vi "FPGA_main.vi"() -> ()   [LabVIEW 2016]
uses:
  <vilib>/Platform/TimedLoop/XDataNode/timing_clust.ctl
  <vilib>/Platform/TimedLoop/XDataNode/nitl_modes.ctl
  <vilib>/Platform/TimedLoop/XDataNode/wakeup.ctl
  FPGA_states.ctl
  <vilib>/rvi/Emulation/niFpgaSctlEmulationGetInTimedLoop.vi
  <vilib>/rvi/Emulation/niFpgaEmulationReportErrorSimple.vi
  <vilib>/rvi/Emulation/niFpgaGetClockAttributes.vi
  <vilib>/rvi/Emulation/niFpgaCriticalErrorInLSC.vi
  <vilib>/rvi/interface/RandomDataEmulation/niFpgaRandomDataHandleErrors.vi
  <vilib>/Platform/TimedLoop/XDataNode/XDataNode.xnode
  <vilib>/rvi/DataTransferAndStorage/Container/XNode/niFpgaContainer.xnode
  <vilib>/rvi/interface/RandomDataEmulation/nirviRandomDataFpgaReadWriteTemplate.vi
  <vilib>/Platform/TimedLoop/XDataNode/XDNodeRunTimeDep.lvlib
  <instrlib>/_niInstr/Basic Elements/v1/FPGA/niInstr Basic Elements v1 FPGA.lvlib
panel:
  in  "BatchSize":u64
  in  "StartTransfer":bool
  out "Count":u64
  out "Iteration":i32
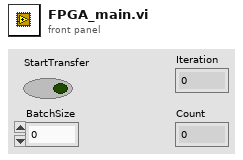
[diagram p1: front panel]
types:
  T1 = typedef "FPGA_states.ctl" = enum16{"Idle", "Flush_FIFO", "CountUp&Transfer"}
  T2 = typedef "XDNodeRunTimeDep.lvlib/timing_clust.ctl" = cluster{"Expected End [f-1]":u64, "Actual End [f-1]":u64, "Finished Late? [f-1]":bool, "Expected End [i-1]":u64, "Actual End [i-1]":u64, "Finished Late? [i-1]":bool, "Expected Start [i]":u64, "Actual Start [i]":u64, "Expected Start [f]":u64, "Actual Start [f]":u64, "Source Name":string, "Structure Name":string, "Period":i64, "Deadline":i64, "Offset":i64, "Start":i64, "Priority":i32, "Timeout":i32, "Mode":T3, "Wakeup Reason":T4, "Error":errorcluster, "Source Type":string, "Secondary Source Type":string, "Global End Time":u64, "Global Start Time":u64, "Frame Duration":u64, "Iteration Duration":u64, "Assigned CPU":i32, "I/O Scan Engine Mode":u32}
  T3 = typedef "XDNodeRunTimeDep.lvlib/nitl_modes.ctl" = enum32{"No Change", "Process missed periods, maintain original phase", "Discard missed periods, maintain original phase", "Process missed periods, ignore original phase", "Discard missed periods, ignore original phase"}
  T4 = typedef "XDNodeRunTimeDep.lvlib/wakeup.ctl" = enum32{"Normal", "Aborted", "Asynchronous wakeup", "Timing source error", "Timed loop error", "Timeout"}
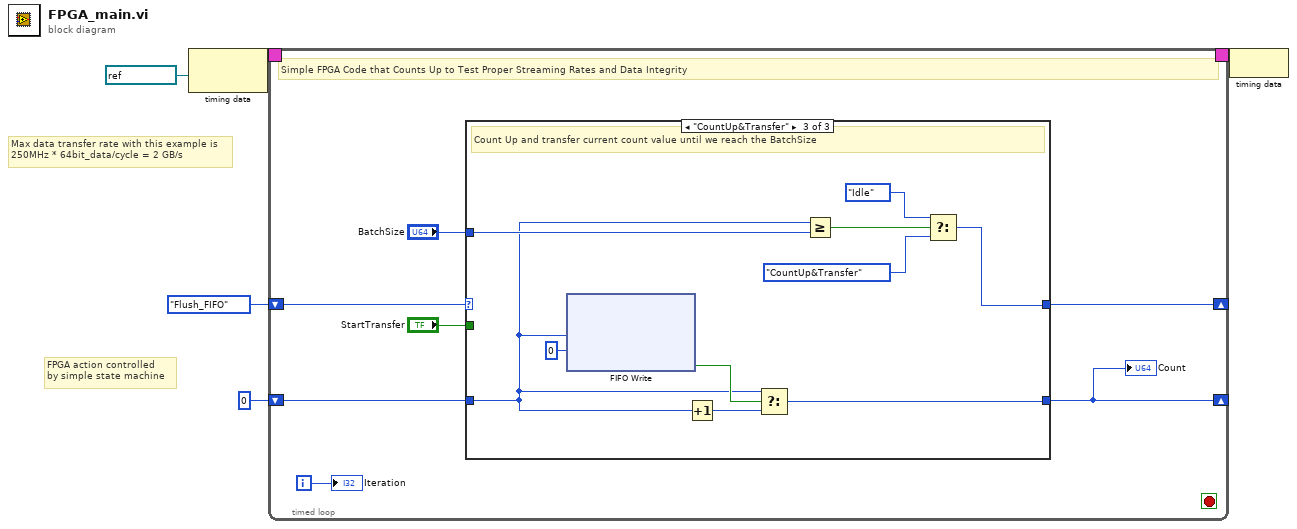
[diagram p0: block diagram]
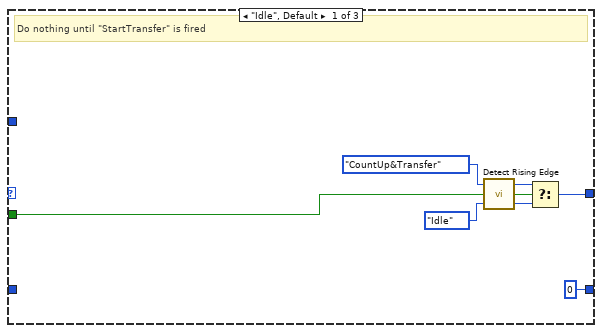
[diagram p2: hidden frame]
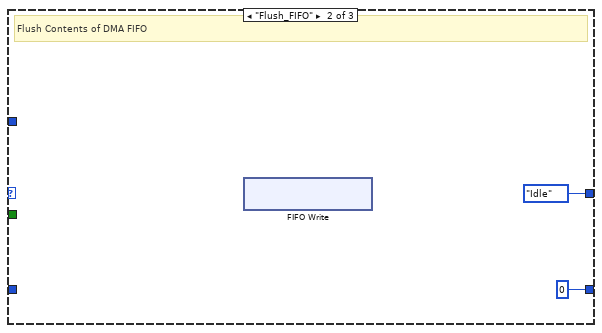
[diagram p3: hidden frame]
diagram:
  # "Max data transfer rate with this example is\n250MHz * 64bit_data/cycle = 2 GB/s"
  # "FPGA action controlled\nby simple state machine"
  n1 = node-c288(refnum<k21> "250MHz" ("Source Name")) -> (w5:T2)
  n2 = timed-loop {
    timing: w5 -> [_]
    timing-out: [_] -> w4
    shift-right: [w11] -> _
    shift-left: u64 0 ("Count") -> [w8]
    shift-right: [w9] -> _
    shift-left: FPGA_states."Flush_FIFO" -> [w10]
    i -> [w12]
    stop <- _ stop-if-true
    # "Simple FPGA Code that Counts Up to Test Proper Streaming Rates and Data Integrity"
    n3 = case shown="\"CountUp&Transfer\"" w10 {
      tunnel: [u64 0 ("Count") u64 0 ("Count") w30] -> w11
      tunnel: [w14 FPGA_states."Idle" w26] -> w9
      tunnel: w8 -> [_ _ w21]
      tunnel: "BatchSize" -> [_ _ w24]
      tunnel: "StartTransfer" -> [w13 _ _]
      frame "Idle", Default {
        # "Do nothing until \"StartTransfer\" is fired"
        n4 = call <instrlib>:"Detect Rising Edge.vi"("signal"=w13) -> ("edge detected"=w16:bool)  [unwired: 14 in]
        n5 = Select(t=FPGA_states."CountUp&Transfer", s=w16, f=FPGA_states."Idle") -> (s? t:f=w14:T1)
      }
      frame "Flush_FIFO" {
        # "Flush Contents of DMA FIFO"
        n6 = xnode "FIFO Write"() -> ()  [unwired: 1 in, 1 out]
      }
      frame "CountUp&Transfer" {
        # "Count Up and transfer current count value until we reach the BatchSize"
        n7 = xnode "FIFO Write"("Element"=w21, "Timeout"=0) -> ("Timed Out?"=w23:bool)  [unwired: 1 in, 1 out]
        n8 = Increment(x=w21) -> (x+1=w22:u64)
        n9 = Select(t=w21, s=w23, f=w22) -> (s? t:f=w30:u64)
        n10 = Greater Or Equal?(x=w21, y=w24) -> (x >= y?=w29:bool)
        n11 = Select(t=FPGA_states."Idle", s=w29, f=FPGA_states."CountUp&Transfer") -> (s? t:f=w26:T1)
      }
    }
    "Count" <- w11
    "Iteration" <- w12
  }
  n12 = node-c288(w4) -> ()
